vi "Hexapod1check.vi"(10 "zpos::1":dbl, 11 "ypos::1":dbl) -> (3 "sdfsdfs":enum16{"guiding", "fiber ref", "Unknown"}(ring))   [LabVIEW 2020]
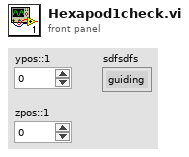
[diagram p1: front panel]
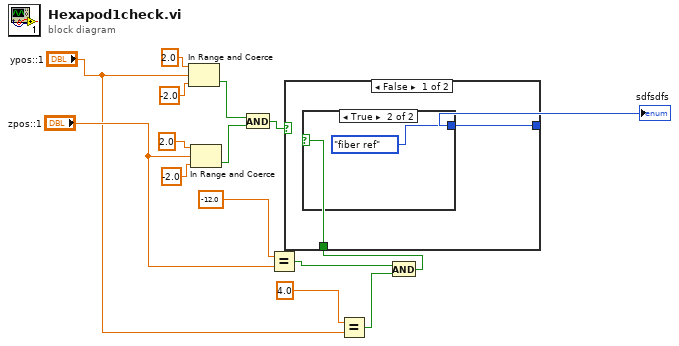
[diagram p0: block diagram]
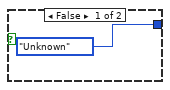
[diagram p2: hidden frame]
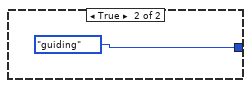
[diagram p3: hidden frame]
diagram:
  n1 = In Range and Coerce(upper limit=2.0, x="ypos::1", lower limit=-2.0) -> (In Range?=w12:bool)  [unwired: 1 out]
  n2 = In Range and Coerce(upper limit=2.0, x="zpos::1", lower limit=-2.0) -> (In Range?=w13:bool)  [unwired: 1 out]
  n3 = And(x=w12, y=w13) -> (x .and. y?=w14:bool)
  n4 = Equal?(x=-12.0 ("lower limit"), y="zpos::1") -> (x = y?=w2:bool)
  n5 = Equal?(x=4.0 ("lower limit"), y="ypos::1") -> (x = y?=w3:bool)
  n6 = And(x=w2, y=w3) -> (x .and. y?=w1:bool)
  n7 = case shown="False" w14 {
    tunnel: [w16 enum16{"guiding", "fiber ref", "Unknown"}."guiding" ("sdfsdfs")] -> w15
    tunnel: w1 -> [w17 _]
    frame False {
      n8 = case shown="True" w17 {
        tunnel: [enum16{"guiding", "fiber ref", "Unknown"}."Unknown" ("sdfsdfs") enum16{"guiding", "fiber ref", "Unknown"}."fiber ref" ("sdfsdfs")] -> w16
        frame False {
        }
        frame True {
        }
      }
    }
    frame True {
    }
  }
  "sdfsdfs" <- w15
